vi "Write Float.vi"(7 "Section":string, 8 "error in":errorcluster, 9 "Value":dbl, 10 "Key":string, 11 "config-base in":refnum<class "config-base.lvclass">) -> (0 "error out":errorcluster, 3 "config-base out":refnum<class "config-base.lvclass">)   [LabVIEW 2020, in "hse-config.lvlib" / "config-base.lvclass"]
doc: "Set a float config key.\n\n____\nHAMPEL SOFTWARE ENGINEERING v3.8.0 (2023-12-18 14:41)"
uses:
  config-base.lvclass
  config-base.lvclass/config-base.ctl
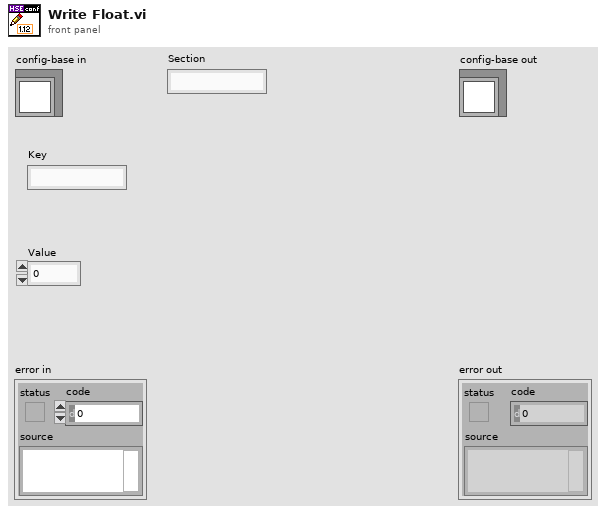
[diagram p1: front panel]
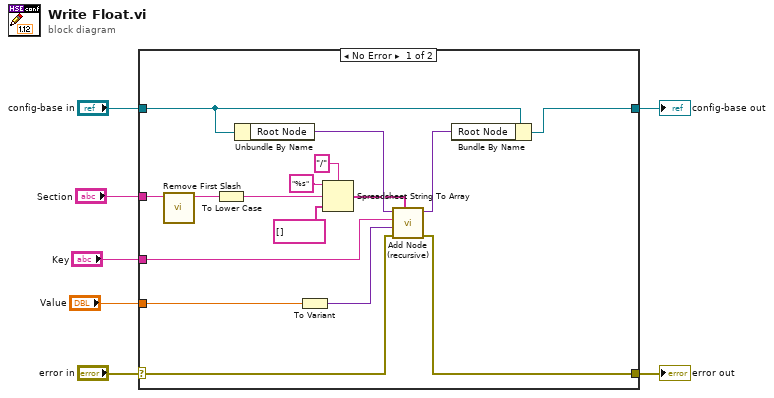
[diagram p0: block diagram]
diagram:
  n1 = case shown="No Error" "error in" {
    selector: "error in" -> [w15 w25]
    tunnel: [w14 w25] -> w6
    tunnel: [w18 w24] -> w4
    tunnel: "config-base in" -> [w20 w24]
    tunnel: "Section" -> [w17 _]
    tunnel: "Key" -> [w12 _]
    tunnel: "Value" -> [w19 _]
    frame No Error {
      n2 = call "Remove First Slash.vi"("Section"=w17) -> ("result string"=w16:string)  [unwired: 10 in]
      n3 = To Lower Case(string=w16) -> (all lower case string=w8:string)
      n4 = Unbundle By Name(w20) -> ("Root Node"=w11:variant)
      n5 = To Variant(anything=w19) -> (Variant=w13:variant)
      n6 = Spreadsheet String To Array(delimiter (Tab)="/" ("Split Pattern"), format string="%s", spreadsheet string=w8, array type (2D Dbl)=string[] []) -> (array=w10:string[])
      n7 = call "Add Node (recursive).vi"("Section"=w10, "error in"=w15, "Value"=w13, "Key"=w12, "Node in"=w11) -> ("error out"=w14:errorcluster, "Node out"=w9:variant)  [unwired: 5 in]
      n8 = Bundle By Name(cluster=w20, "Root Node"=w9) -> (w18:refnum<class "config-base.lvclass">)
    }
    frame Error {
    }
  }
  "error out" <- w6
  "config-base out" <- w4
